vi "FittingAlg.vi"(0 "Pos":dbl[](array[numeric]), 1 "Cal px/V":dbl=1.0 format="%#_13g", 5 "initial parameters":dbl[](array[numeric]), 9 "Volt":dbl[](array[numeric]), 12 "Boolean in":bool, 13 "Offset":sgl) -> (3 "error":i32, 4 "best fit parameters":dbl[](array[numeric]), 6 "Boolean out":bool, 10 "residue":dbl, 15 "error out":errorcluster)   [LabVIEW 2019]
uses:
  <vilib>/Analysis/3filter.llb/Savitzky-Golay Filter (DBL).vi
  <vilib>/ptbypt/NI_PtbyPt.lvlib
  <vilib>/Analysis/NI_AALBase.lvlib
  <vilib>/gmath/NI_Gmath.lvlib
  <vilib>/gmath/NumericalOptimization/Nonlinear Curve Fit LM formula string.vi
  <vilib>/Analysis/NI_AALPro.lvlib
panel:
  out "XY Graph":T1(graph)
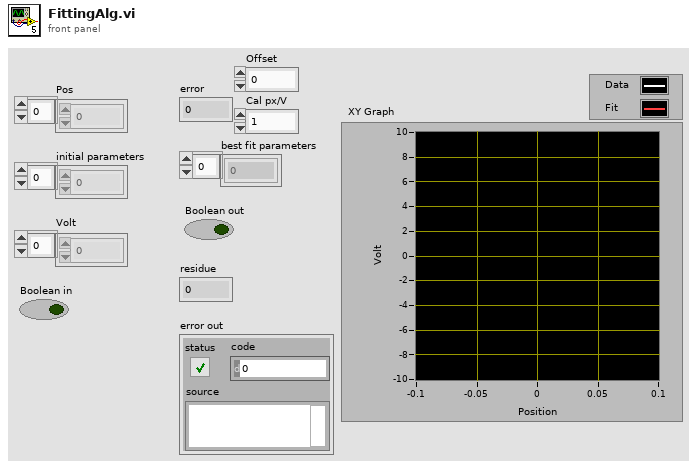
[diagram p1: front panel]
types:
  T1 = cluster{"Filtered X":dbl[], "best nonlinear fit":dbl[]}[]
  T2 = cluster{"model":string, "Parameters":string[], "x":string}
  T3 = cluster{"Filtered X":dbl[], "Best Polynomial Fit":dbl[]}
  T4 = cluster{"Filtered X":dbl[], "Best Polynomial Fit":dbl[]}[]
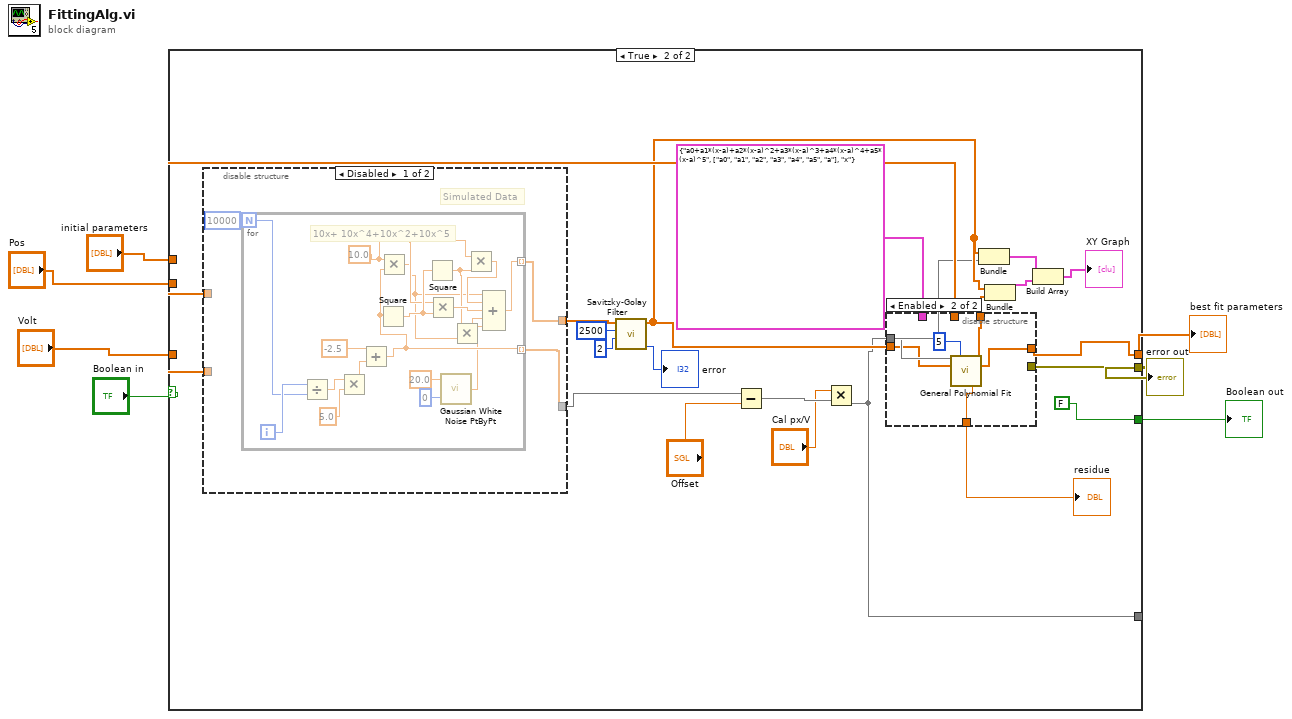
[diagram p0: block diagram]
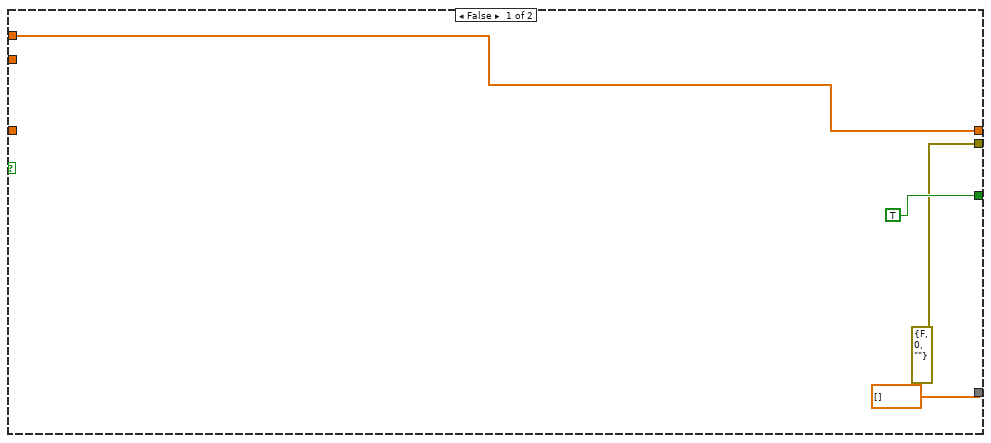
[diagram p2: hidden frame]
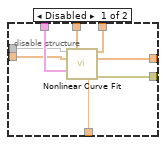
[diagram p3: hidden frame]
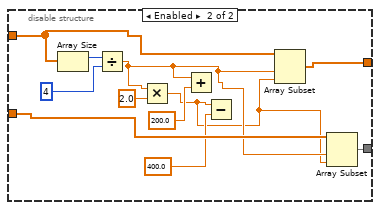
[diagram p4: hidden frame]
diagram:
  n1 = case shown="True" "Boolean in" {
    tunnel: [w11 w14] -> w6
    tunnel: [TRUE FALSE] -> w3
    tunnel: "initial parameters" -> [w11 w24]
    tunnel: [errorcluster {"status"=FALSE, "code"=0, "source"=""} ("error out") w31] -> w7
    tunnel: "Volt" -> [_ w30]
    tunnel: "Pos" -> [_ w29]
    tunnel: [dbl[] [] w13] -> _
    frame False {
    }
    frame True {
      n2 = disable-structure shown="Disabled" {
        disable-tunnel: [w49 w74] -> w33
        disable-tunnel: [w48 w73] -> w22
        disable-tunnel: w29 -> [_ w79]
        disable-tunnel: w30 -> [_ w76]
        frame Disabled {
          # "Simulated Data"
          n3 = for {
            N: 10000 -> [w66]
            tunnel: [w63] -> w48 mode=indexing
            tunnel: [w57] -> w49 mode=indexing
            i -> [w67]
            w61 = 10.0
            # "10x+ 10x^4+10x^2+10x^5"
            n4 = Divide(x=w67, y=w66) -> (x/y=w65:dbl)
            n5 = Multiply(x=w65, y=5.0) -> (x*y=w56:dbl)
            n6 = Add(x=-2.5, y=w56) -> (x+y=w63:dbl)
            n7 = Square(x=w63) -> (x^2=w62:dbl)
            n8 = Multiply(x=w61, y=w63) -> (x*y=w51:dbl)
            n9 = Square(x=w62) -> (x^2=w52:dbl)
            n10 = Multiply(x=w61, y=w62) -> (x*y=w60:dbl)
            n11 = call <vilib>:"Gaussian White Noise PtByPt.vi"("seed"=0, "standard deviation"=20.0) -> ("Gaussian white noise"=w53:dbl)  [unwired: 1 in]
            n12 = Multiply(x=w52, y=w51) -> (x*y=w58:dbl)
            n13 = Multiply(x=w61, y=w52) -> (x*y=w59:dbl)
            n14 = Compound Arithmetic op=ADD(w51, w59, w60, w58, w53) -> (w57:dbl)
          }
        }
        frame Enabled {
          n15 = Array Size(array=w79) -> (size(s)=w78:i32)
          n16 = Divide(x=w78, y=4 ("index")) -> (x/y=w70:dbl)
          n17 = Multiply(x=w70, y=2.0) -> (x*y=w69:dbl)
          n18 = Add(x=w70, y=200.0) -> ()  [unwired: 1 out]
          n19 = Subtract(x=w69, y=400.0) -> ()  [unwired: 1 out]
          n20 = Array Subset(array=w79, index=w70, length=w69) -> (w74:dbl[])
          n21 = Array Subset(array=w76, index=w70, length=w69) -> (w73:dbl[])
        }
      }
      n22 = call-poly <vilib>:"Savitzky-Golay Filter.vi"("polynomial order"=2, "side points"=2500, "X"=w33) -> ("error"=→"error":i32, "Filtered X"=w20:dbl[])  [unwired: 7 in]
      n23 = Subtract(x=w22, y="Offset") -> (x-y=w15:dbl[])
      n24 = Multiply(x="Cal px/V", y=w15) -> (x*y=w13:dbl[])
      n25 = disable-structure shown="Enabled" {
        disable-tunnel: [w41 _] -> w31
        disable-tunnel: T2 {"model"="a0+a1*(x-a)+a2*(x-a)^2+a3*(x-a)^3+a4*(x-a)^4+a5*(x-a)^5", "Parameters"=["a0", "a1", "a2", "a3", "a4", "a5", "a"], "x"="x"} ("model description") -> [w40 _]
        disable-tunnel: w24 -> [w39 _]
        disable-tunnel: [w38 w42] -> w21
        disable-tunnel: w20 -> [w37 w46]
        disable-tunnel: [w36 w45] -> w16
        disable-tunnel: [w35 w43] -> w14
        disable-tunnel: w13 -> [w34 w47]
        frame Disabled {
          n26 = call-poly <vilib>:"Nonlinear Curve Fit.vi"("Y"=w34, "initial parameters"=w39, "X"=w37, "model description"=w40) -> ("best nonlinear fit"=w38:dbl[], "best fit parameters"=w35:dbl[], "residue"=w36:dbl, "error out"=w41:errorcluster)  [unwired: 7 in, 1 out]
        }
        frame Enabled {
          n27 = call <vilib>:"General Polynomial Fit.vi"("Y"=w47, "polynomial order"=5, "X"=w46) -> ("Best Polynomial Fit"=w42:dbl[], "Polynomial Coefficients"=w43:dbl[], "residue"=w45:dbl)  [unwired: 9 in, 1 out]
        }
      }
      "residue" <- w16
      n28 = Bundle("Filtered X"=w20, w13) -> (w19:cluster{"Filtered X":dbl[], dbl[]})  [unwired: 1 in]
      n29 = Bundle("Filtered X"=w20, "Best Polynomial Fit"=w21) -> (w18:T3)  [unwired: 1 in]
      n30 = Build Array(w19, w18) -> (→"XY Graph":T4)
    }
  }
  "error out" <- w7
  "best fit parameters" <- w6
  "Boolean out" <- w3
